vi "ConfigureDlg.vi"(8 "error in (no error)":errorcluster, 11 "NISTFGenPluginsBase in":refnum<class "NISTFGenPluginsBase.lvclass">) -> (0 "error out":errorcluster, 3 "NISTFGenPluginsBase out":refnum<class "NISTFGenPluginsBase.lvclass">)   [LabVIEW 2014, in "FGenPlugins.lvlib" / "NISTFGenPluginsBase.lvclass"]
uses:
  NISTFGenPluginsBase.lvclass
  TypeDef/TriggerParams.ctl
  TypeDef/ChannelParamElement.ctl
  <userlib>/NIST/BaseClasses/BasePlugin_class/BasePlugin.lvclass/BasePlugin.ctl
  <userlib>/NIST/BaseClasses/BasePlugin_class/Accessors/Read PluginIniFilePath.vi
  <vilib>/Utility/config.llb/NI_LVConfig.lvlib
panel:
  in  "btnCancel":bool
  in  "btnDone":bool
  in  "dSampleRate":dbl caption="Sample Rate"
  in  "ChannelParams":T1[](array[typedef]) caption="Channels" {"eOutputMode" items=["Function", "Arbitrary", "Sequence"]; "eOperateMode" items=["Continuous", "Burst"]}
  in  "TriggerParams":T2={"eTrigger"=0, "eEdge"=10280, "sSource"=""} caption="Trigger" {"eEdge" items=["Rising"=10280, "Falling"=10171]; "eTrigger" items=["None", "Digital", "Analog"]}
  in  "eRefClk":u16(ring) caption="Reference Clock" items=["Internal", "External", "RTSI"]
  in  "Handle":string
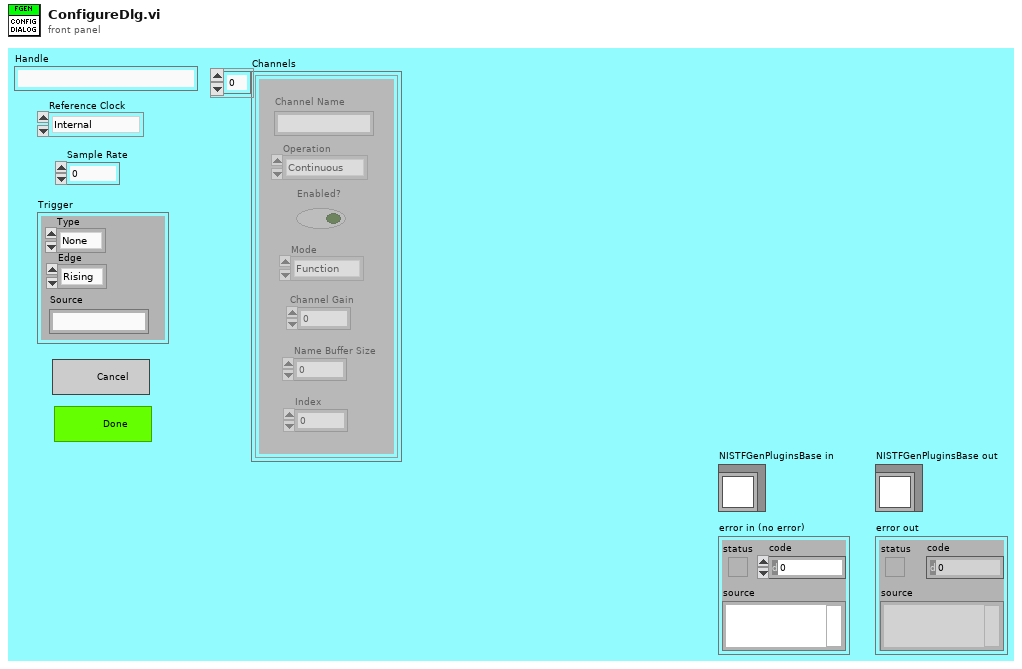
[diagram p1: front panel]
types:
  T1 = typedef "FGenPlugins.lvlib/NISTFGenPluginsBase.lvclass/ChannelParamElement.ctl" = cluster{"sName":string, "eOperateMode":u16, "bEnabled":bool, "eOutputMode":u16, "iIndex":i32, "iNameBufferSize":i32, "fGain":dbl}
  T2 = typedef "FGenPlugins.lvlib/NISTFGenPluginsBase.lvclass/TriggerParams.ctl" = cluster{"eTrigger":u16, "eEdge":u16, "sSource":string}
  T3 = enum32{"Invalid", "Default", "Floating", "Floating/Auto-Hide", "Modal"}
  T4 = typedef "FGenPlugins.lvlib/NISTFGenPluginsBase.lvclass/ArbWfrmParams.ctl" = cluster{"sWfrmHandle":string, "iSize":i32, "dData":dbl[], "dGain":dbl, "dOffset":dbl, "dSampleRate":dbl}
  T5 = typedef "FGenPlugins.lvlib/NISTFGenPluginsBase.lvclass/StdWaveformParams.ctl" = cluster{"eWaveform":u16, "dAmplitude":dbl, "dDcOffset":dbl, "dFrequency":dbl, "dStartPhase":dbl, "dSampleRate":dbl, "dNumSamples":dbl}
  T6 = typedef "NI_LVConfig.lvlib/Config Data RefNum.ctl" = refnum<k1>
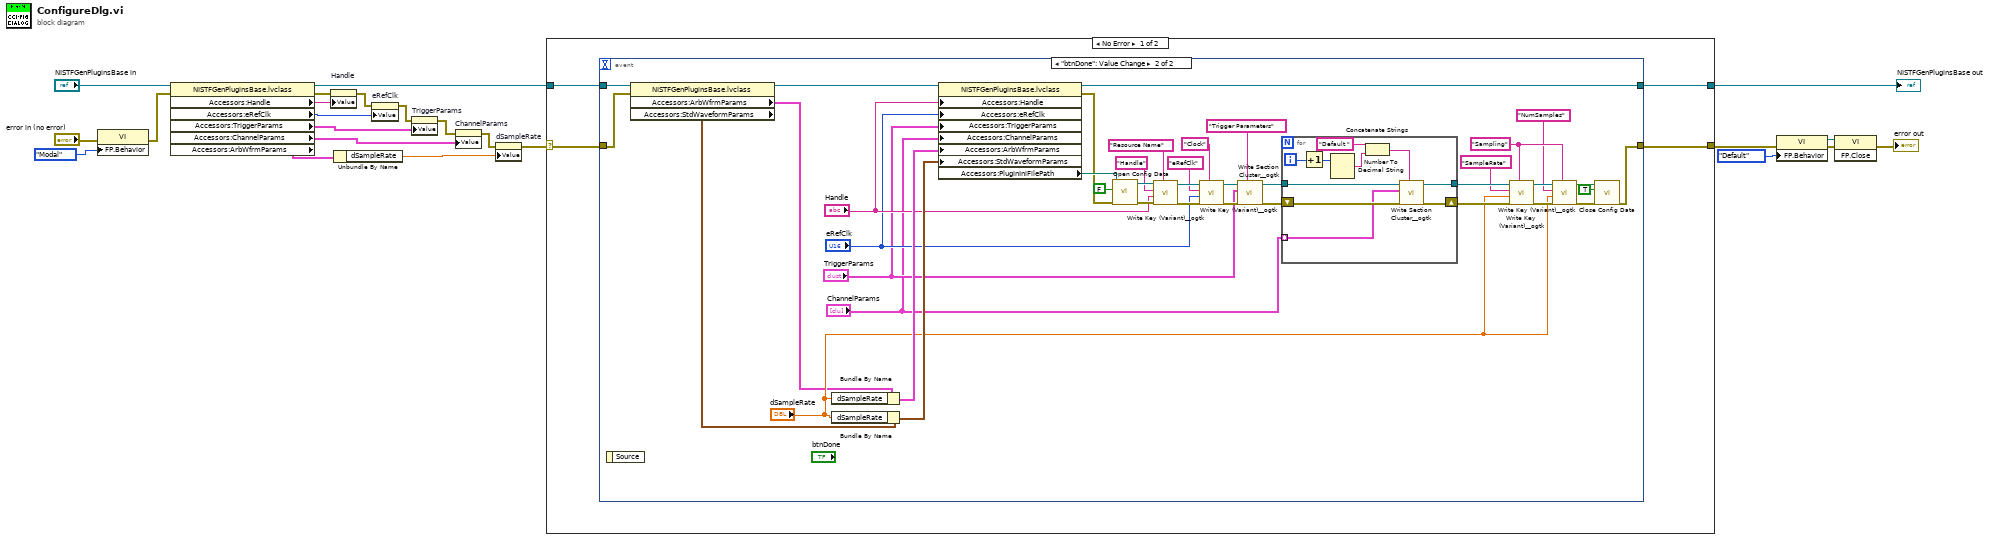
[diagram p0: block diagram]
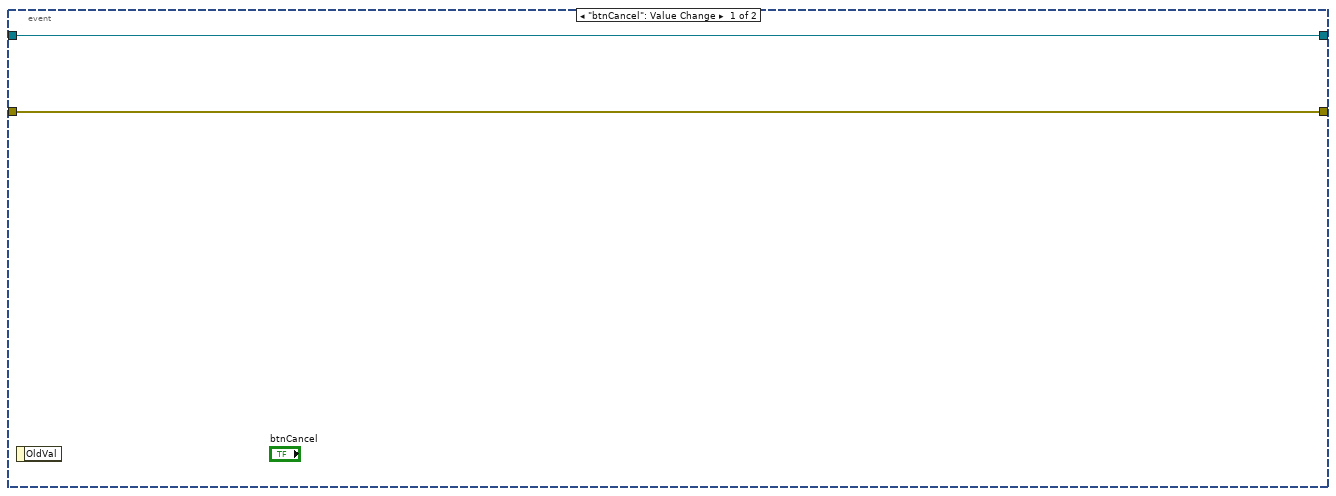
[diagram p2: hidden frame]
diagram:
  n1 = property class="VI"(error in="error in (no error)", "FP.Behavior"=T3."Modal" ("Front Panel Window:Behavior")) -> (error out=w18:errorcluster)  [unwired: 1 in, 1 out]
  n2 = property class="NISTFGenPluginsBase.lvclass"(reference="NISTFGenPluginsBase in", error in=w18) -> (reference out=w19:refnum<class "NISTFGenPluginsBase.lvclass">, error out=w16:errorcluster, "Accessors:Handle"=w17:string, "Accessors:eRefClk"=w15:u16, "Accessors:TriggerParams"=w13:T2, "Accessors:ChannelParams"=w11:T1[], "Accessors:ArbWfrmParams"=w9:T4)
  n3 = property on="Handle" class="Str"(error in=w16, "Value"=w17) -> (error out=w14:errorcluster)  [unwired: 1 in, 1 out]
  n4 = Unbundle By Name(w9) -> ("dSampleRate"=w8:dbl)
  n5 = property on="eRefClk" class="Ring (strict)"(error in=w14, "Value"=w15) -> (error out=w12:errorcluster)  [unwired: 1 in, 1 out]
  n6 = property on="TriggerParams" class="Clust (strict)"(error in=w12, "Value"=w13) -> (error out=w10:errorcluster)  [unwired: 1 in, 1 out]
  n7 = property on="ChannelParams" class="Arr (strict)"(error in=w10, "Value"=w11) -> (error out=w7:errorcluster)  [unwired: 1 in, 1 out]
  n8 = property on="dSampleRate" class="DigNum (strict)"(error in=w7, "Value"=w8) -> (error out=w6:errorcluster)  [unwired: 1 in, 1 out]
  n9 = case shown="No Error" w6 {
    selector: w6 -> [w25 w80]
    tunnel: [w26 w81] -> w22
    tunnel: w19 -> [w27 w81]
    tunnel: [w24 w80] -> w5
    frame No Error {
      n10 = event shown="[1] \"btnDone\": Value Change" {
        selector: _ -> [_ _]
        dyn-events: _ -> [_ _]
        timeout: _ -> [_ _]
        tunnel: w27 -> [w29 w69]
        tunnel: [w29 w34] -> w26
        tunnel: [w28 w35] -> w24
        tunnel: w25 -> [w28 w32]
        event "btnCancel": Value Change {
          n11 = event-data() -> ()  [unwired: 1 in, 1 out]
        }
        event "btnDone": Value Change {
          w41 = "Sampling" ("section")
          n12 = event-data() -> ()  [unwired: 1 in, 1 out]
          n13 = property class="NISTFGenPluginsBase.lvclass"(reference=w69, error in=w32) -> (reference out=w33:refnum<class "NISTFGenPluginsBase.lvclass">, "Accessors:ArbWfrmParams"=w31:T4, "Accessors:StdWaveformParams"=w30:T5)  [unwired: 1 out]
          n14 = Bundle By Name(cluster=w31, "dSampleRate"="dSampleRate") -> (w68:T4)
          n15 = Bundle By Name(cluster=w30, "dSampleRate"="dSampleRate") -> (w67:T5)
          n16 = property class="NISTFGenPluginsBase.lvclass"(reference=w33, "Accessors:Handle"="Handle", "Accessors:eRefClk"="eRefClk", "Accessors:TriggerParams"="TriggerParams", "Accessors:ChannelParams"="ChannelParams", "Accessors:ArbWfrmParams"=w68, "Accessors:StdWaveformParams"=w67) -> (reference out=w34:refnum<class "NISTFGenPluginsBase.lvclass">, error out=w65:errorcluster, "Accessors:PluginIniFilePath"=w66:path)  [unwired: 1 in]
          n17 = call <vilib>:"Open Config Data.vi"("error in (no error)"=w65, "create file if necessary (T)"=FALSE, "configuration file path"=w66) -> ("error out"=w63:errorcluster, "refnum"=w62:T6)  [unwired: 6 in, 1 out]
          n18 = call <userlib>:"Write Key (Variant)__ogtk.vi"("section"="Resource Name", "error in (no error)"=w63, "key-value"="Handle", "key (optional)"="Handle", "refnum"=w62) -> ("error out"=w58:errorcluster, "refnum out"=w57:T6)  [unwired: 5 in]
          n19 = call <userlib>:"Write Key (Variant)__ogtk.vi"("section"="Clock", "error in (no error)"=w58, "key-value"="eRefClk", "key (optional)"="eRefClk", "refnum"=w57) -> ("error out"=w53:errorcluster, "refnum out"=w52:T6)  [unwired: 5 in]
          n20 = call <userlib>:"Write Section Cluster__ogtk.vi"("section (optional)"="Trigger Parameters", "error in (no error)"=w53, "Section Formatted Cluster"="TriggerParams", "refnum"=w52) -> ("error out"=w48:errorcluster, "dup refnum"=w47:T6)  [unwired: 6 in]
          n21 = for {
            tunnel: "ChannelParams" -> [w72] mode=indexing
            shift-right: [w71] -> w45
            shift-left: w48 -> [w73]
            tunnel: w47 -> [w75]
            tunnel: [w70] -> w46
            i -> [w79]
            n22 = Increment(x=w79) -> (x+1=w78:i32)
            n23 = Number To Decimal String(number=w78) -> (decimal integer string=w77:string)  [unwired: 1 in]
            n24 = Concatenate Strings("Default " ("string"), w77) -> (w74:string)
            n25 = call <userlib>:"Write Section Cluster__ogtk.vi"("section (optional)"=w74, "error in (no error)"=w73, "Section Formatted Cluster"=w72, "refnum"=w75) -> ("error out"=w71:errorcluster, "dup refnum"=w70:T6)  [unwired: 6 in]
          }
          n26 = call <userlib>:"Write Key (Variant)__ogtk.vi"("section"=w41, "error in (no error)"=w45, "key-value"="dSampleRate", "key (optional)"="SampleRate", "refnum"=w46) -> ("error out"=w43:errorcluster, "refnum out"=w42:T6)  [unwired: 5 in]
          n27 = call <userlib>:"Write Key (Variant)__ogtk.vi"("section"=w41, "error in (no error)"=w43, "key-value"="dSampleRate", "key (optional)"="NumSamples", "refnum"=w42) -> ("error out"=w38:errorcluster, "refnum out"=w37:T6)  [unwired: 5 in]
          n28 = call <vilib>:"Close Config Data.vi"("error in (no error)"=w38, "write file if changed (T)"=TRUE, "refnum"=w37) -> ("error out"=w35:errorcluster)  [unwired: 7 in, 1 out]
        }
      }
    }
    frame Error {
    }
  }
  "NISTFGenPluginsBase out" <- w22
  n29 = property class="VI"(error in=w5, "FP.Behavior"=T3."Default" ("Front Panel Window:Behavior")) -> (reference out=w2:refnum<vi>, error out=w4:errorcluster)  [unwired: 1 in]
  n30 = invoke class="VI" method="FP.Close"(reference=w2, error in=w4) -> (error out=→"error out":errorcluster)  [unwired: 1 in, 2 out]
